vi "Get Fields.vi"(11 "File Info in":refnum<class "File Info.lvclass">) -> (2 "Fields":variant[](array[variant]), 3 "File Info out":refnum<class "File Info.lvclass">)   [LabVIEW 2019, in "Electronic Datasheet.lvlib" / "File Info.lvclass"]
uses:
  File Info.lvclass
  File Info.lvclass/File Info.ctl
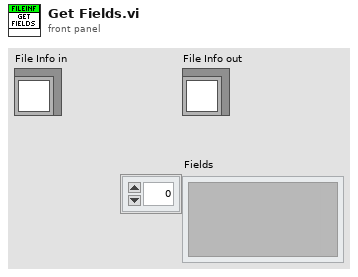
[diagram p1: front panel]
types:
  T1 = cluster{"FileName":string, "FileVersion":u8, "FileRevision":u8, "EDSVersion":string, "Description":string, "CreationTime":string, "CreationDate":string, "CreatedBy":string, "ModificationTime":string, "ModificationDate":string, "ModifiedBy":string}
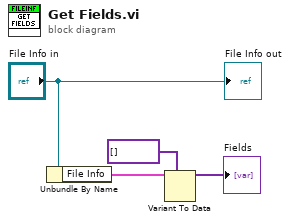
[diagram p0: block diagram]
diagram:
  n1 = Unbundle By Name("File Info in") -> ("File Info"=w3:T1)
  n2 = Variant To Data(type=variant[] [], Variant=w3) -> (data=→"Fields":variant[])  [unwired: 1 in, 1 out]
  "File Info out" <- "File Info in"
